vi "Update Pin Map.vi"(0 "Pin Map Path":string, 2 "Sequence Context In":refnum<k7>, 3 "error in":errorcluster) -> (10 "error out":errorcluster)   [LabVIEW 2020, in "NIScopeAcquireWaveform.lvlib"]
uses:
  NIScopeAcquireWaveform.lvlib
  <vilib>/MeasurementLink/MeasurementLink Measurement Server/MeasurementLink Measurement Server.lvlib
  <vilib>/MeasurementLink/MeasurementLink Discovery Client/MeasurementLink Discovery Client.lvlib
  <vilib>/MeasurementLink/MeasurementLink Discovery Client/RPC Messages/ni_measurementlink_discovery_v1_ResolveServiceRequest.ctl
  <vilib>/MeasurementLink/MeasurementLink Pin Map Client/MeasurementLink Pin Map Client.lvlib
  <vilib>/MeasurementLink/MeasurementLink Pin Map Client/RPC Messages/ni_measurementlink_pinmap_v1_UpdatePinMapFromXmlRequest.ctl
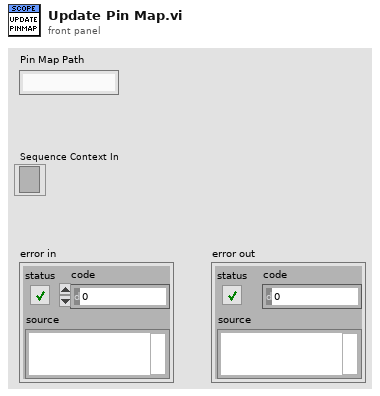
[diagram p1: front panel]
types:
  T1 = typedef "MeasurementLink Pin Map Client.lvlib/ni_measurementlink_pinmap_v1_UpdatePinMapFromXmlRequest.ctl" = cluster{"pin_map_id":string, "pin_map_xml":string}
  T2 = typedef "MeasurementLink Discovery Client.lvlib/ni_measurementlink_discovery_v1_ResolveServiceRequest.ctl" = cluster{"provided_interface":string, "service_class":string}
  T3 = typedef "grpc-lvsupport-release.lvlib/grpcId.ctl" = u64
  T4 = typedef "MeasurementLink Discovery Client.lvlib/ni_measurementlink_discovery_v1_ServiceLocation.ctl" = cluster{"location":string, "insecure_port":string, "ssl_authenticated_port":string}
  T5 = typedef "MeasurementLink Pin Map Client.lvlib/ni_measurementlink_pinmap_v1_PinMap.ctl" = cluster{"pin_map_id":string}
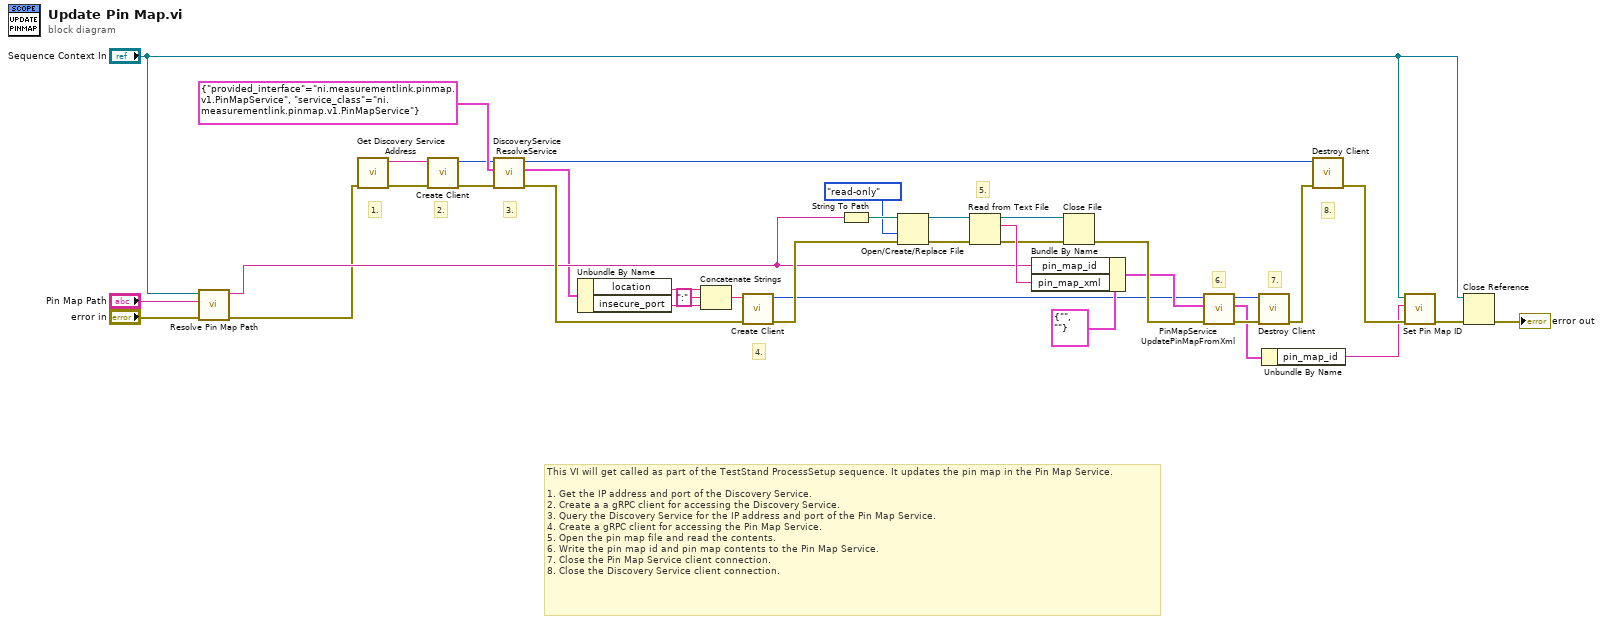
[diagram p0: block diagram]
diagram:
  # "8."
  # "7."
  # "6."
  # "5."
  # "4."
  # "3."
  # "2."
  # "1."
  # "This VI will get called as part of the TestStand ProcessSetup sequence. It updates the pin map in the Pin Map Service. \n\n1. Get the IP address and port of the Discovery Service.\n2. Create a a gRPC client for accessing the Discovery Service.\n3. Query the Discovery Service for the IP address and port of the Pin Map Service.\n4. Create a gRPC client for accessing the Pin Map Service.\n5. Open the pin map file and read the contents.\n6. Write the pin map id and pin map contents to the Pin Map Service.\n7. Close the Pin Map Service client connection.\n8. Close the Discovery Service client connection."
  n1 = call "Resolve Pin Map Path.vi"("error in"="error in", "Pin Map Path"="Pin Map Path", "Sequence Context In"="Sequence Context In") -> ("error out"=w13:errorcluster, "Pin Map Path"=w14:string)  [unwired: 7 in]
  n2 = call <vilib>:"Get Discovery Service Address.vi"("error in"=w13) -> ("error out"=w37:errorcluster, "address"=w36:string)  [unwired: 9 in]
  n3 = call <vilib>:"Create Client.vi"("error in"=w37, "address"=w36) -> ("error out"=w26:errorcluster, "gRPC ID Out"=w34:T3)  [unwired: 8 in]
  n4 = call <vilib>:"DiscoveryService ResolveService.vi"("error in"=w26, "Request Data"=T2 {"provided_interface"="ni.measurementlink.pinmap.v1.PinMapService", "service_class"="ni.measurementlink.pinmap.v1.PinMapService"}, "gRPC ID"=w34) -> ("error out"=w25:errorcluster, "Response Data"=w1:T4, "gRPC ID out"=w16:T3)  [unwired: 6 in]
  n5 = Unbundle By Name(w1) -> ("location"=w3:string, "insecure_port"=w4:string)
  n6 = Concatenate Strings(w3, ":" ("string"), w4) -> (w2:string)
  n7 = call <vilib>:"Create Client.vi"("error in"=w25, "address"=w2) -> ("error out"=w24:errorcluster, "gRPC ID Out"=w20:T3)  [unwired: 8 in]
  n8 = String To Path(string=w14) -> (path=w33:path)
  n9 = Open/Create/Replace File(file path (use dialog)=w33, error in=w24, access (0:read/write)=enum16{"read/write", "read-only", "write-only"}."read-only") -> (refnum out=w30:refnum<file>, error out=w31:errorcluster)  [unwired: 3 in, 1 out]
  n10 = Read from Text File(file (use dialog)=w30, error in=w31) -> (refnum out=w27:refnum<file>, text=w29:string, error out=w28:errorcluster)  [unwired: 2 in, 1 out]
  n11 = Bundle By Name(cluster=T1 {"pin_map_id"="", "pin_map_xml"=""} ("Request Data"), "pin_map_id"=w14, "pin_map_xml"=w29) -> (w21:T1)
  n12 = Close File(refnum=w27, error in=w28) -> (error out=w23:errorcluster)  [unwired: 1 out]
  n13 = call <vilib>:"PinMapService UpdatePinMapFromXml.vi"("error in"=w23, "Request Data"=w21, "gRPC ID"=w20) -> ("error out"=w19:errorcluster, "Response Data"=w15:T5, "gRPC ID out"=w18:T3)  [unwired: 6 in]
  n14 = call <vilib>:"Destroy Client.vi"("error in"=w19, "gRPC ID"=w18) -> ("error out"=w17:errorcluster)  [unwired: 9 in]
  n15 = Unbundle By Name(w15) -> ("pin_map_id"=w7:string)
  n16 = call <vilib>:"Destroy Client.vi"("error in"=w17, "gRPC ID"=w16) -> ("error out"=w12:errorcluster)  [unwired: 9 in]
  n17 = call "Set Pin Map ID.vi"("error in"=w12, "pin_map_id"=w7, "Sequence Context"="Sequence Context In") -> ("error out"=w11:errorcluster)  [unwired: 8 in]
  n18 = Close Reference(reference="Sequence Context In", error in (no error)=w11) -> (error out=→"error out":errorcluster)
